vi "E0_Ecuacion.vi"(1 "b":dbl, 2 "a":dbl) -> (0 "y":dbl)   [LabVIEW 2020]
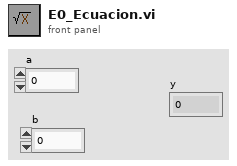
[diagram p1: front panel]
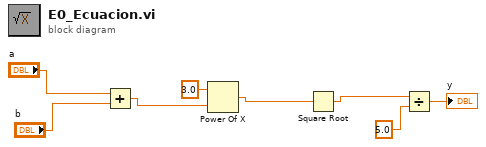
[diagram p0: block diagram]
diagram:
  n1 = Add(x="a", y="b") -> (x+y=w5:dbl)
  n2 = Power Of X(1:w5, 2:3.0 ("y")) -> (0:w3:dbl)
  n3 = Square Root(x=w3) -> (sqrt(x)=w2:dbl)
  n4 = Divide(x=w2, y=5.0) -> (x/y=→"y":dbl)
